vi "box catch.vi"(8 "Error In":errorcluster, 9 "Position in":T4, 11 "main.ctl":T1) -> (0 "Error Out":errorcluster, 1 "Position out":T4, 3 "main.ctl 2":T1={"vision board"={"common room"=[["red", "black", "blue", "", "green"], ["", "", "", "", ""], ["", "", "", "", ""]], "recycle"="NONE"}, "block box"={"block box"=[["", "Black", "", ""], ["", "Red", "", ""], ["Black", "", "", "Blue"]]}, "on robot "=[], "base position"=[], "On robot target"=[]})   [LabVIEW 2019]
uses:
  main data.ctl
  vision/vision_board_ctl.ctl
  block box.ctl
  subVI/move/position cluster.ctl
  box state.ctl
  subVI/move control/move and align/move_cluster.ctl
  servo state.ctl
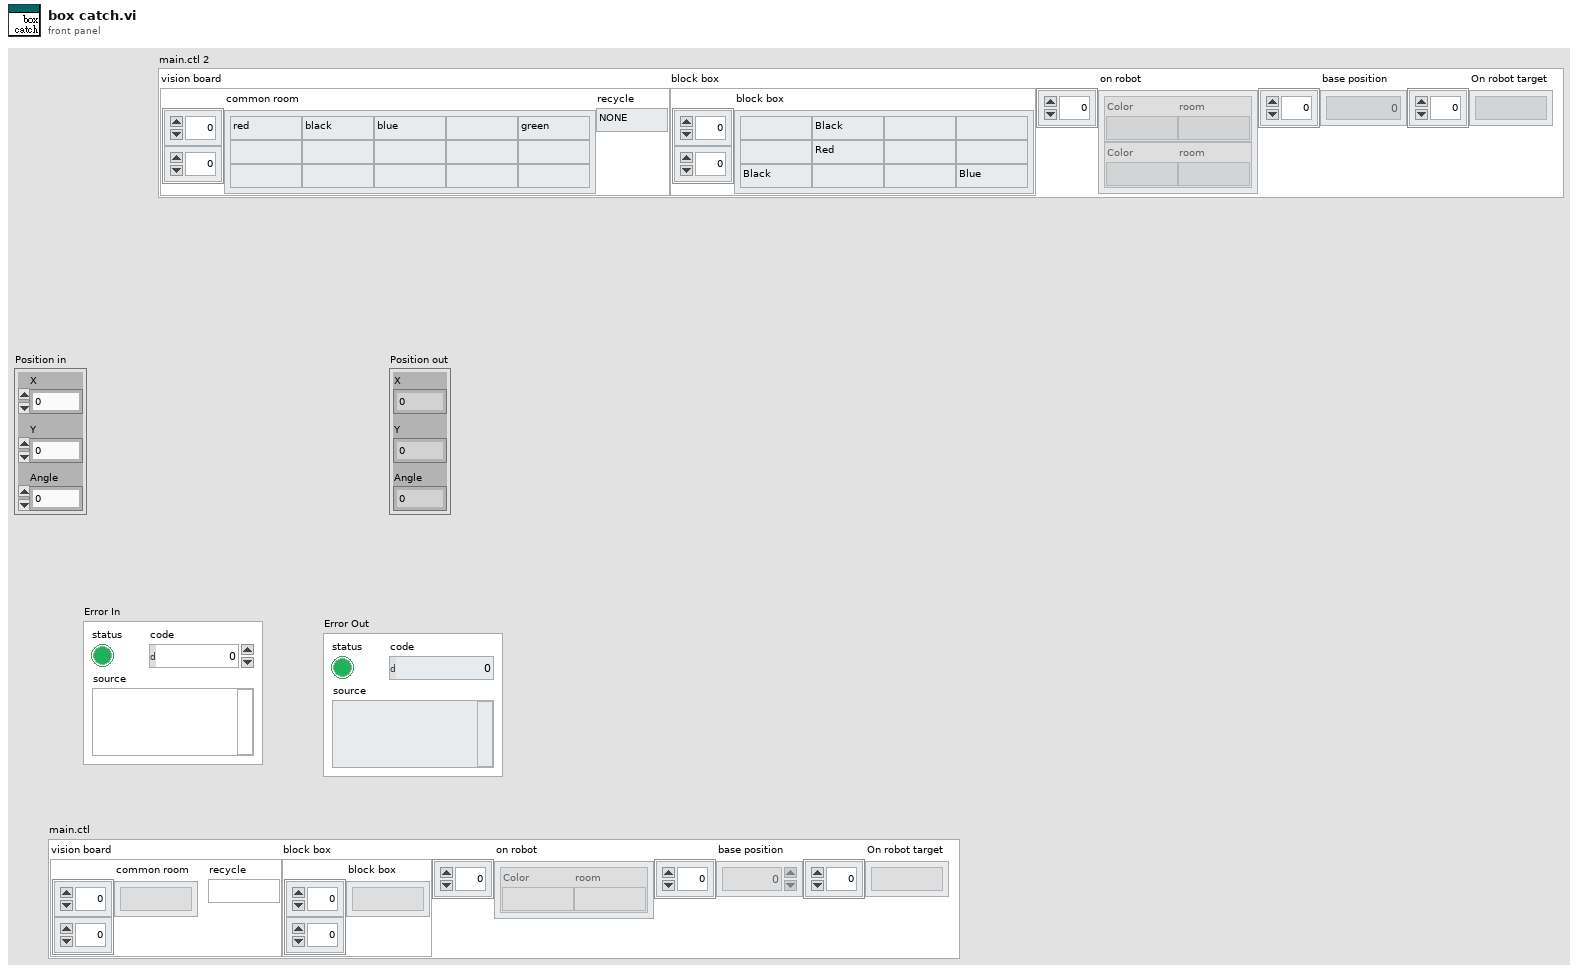
[diagram p1: front panel]
types:
  T1 = typedef "main data.ctl" = cluster{"vision board":T2, "block box":T3, "on robot ":cluster{"Color":string, "room":string}[], "base position":dbl[], "On robot target":string[]}
  T2 = typedef "vision_board_ctl.ctl" = cluster{"common room":string[][], "recycle":string}
  T3 = typedef "block box.ctl" = cluster{"block box":string[][]}
  T4 = typedef "position cluster.ctl" = cluster{"X":dbl, "Y":dbl, "Angle":dbl}
  T5 = typedef "servo state.ctl" = enum16{"catch", "cam-1", "put", "side", "center", "side-2", "put-2"}
  T6 = typedef "move_cluster.ctl" = cluster{"X":dbl, "Y":dbl, "degree":dbl, "speed":dbl}
  T7 = typedef "box state.ctl" = enum16{"init", "vision", "catch"}
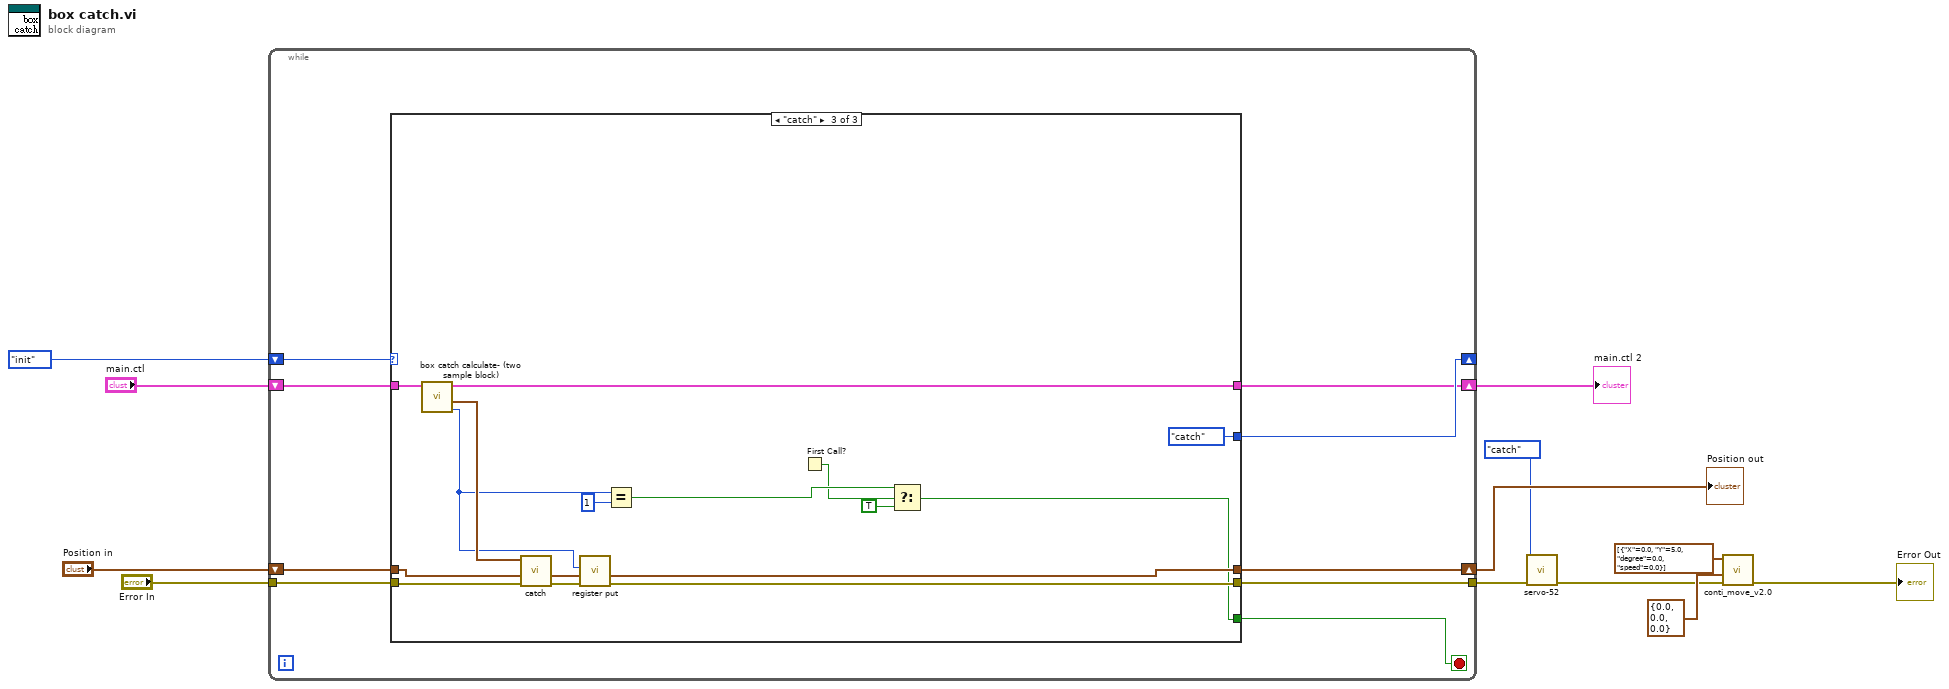
[diagram p0: block diagram]
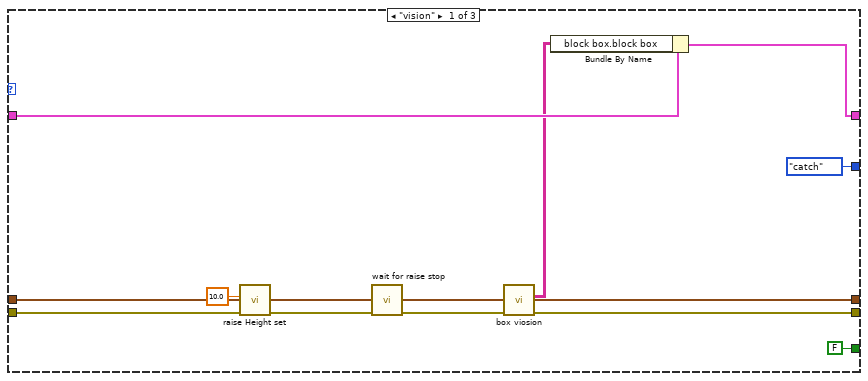
[diagram p2: hidden frame]
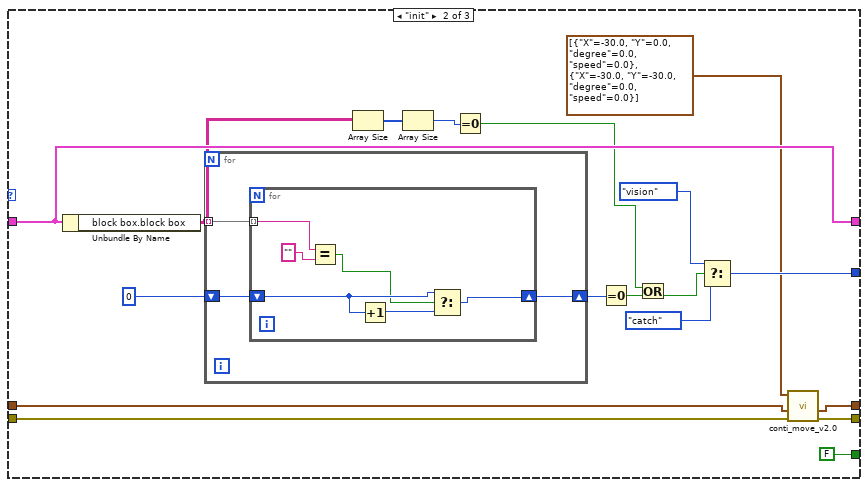
[diagram p3: hidden frame]
diagram:
  n1 = while {
    shift-right: [w19] -> _
    shift-left: box_state."init" -> [w20]
    tunnel: "Error In" -> [w17]
    tunnel: [w16] -> w5
    shift-right: [w13] -> w7
    shift-left: "main.ctl" -> [w21]
    shift-right: [w14] -> w8
    shift-left: "Position in" -> [w15]
    stop <- w18 stop-if-true
    n2 = case shown="\"catch\"" w20 {
      tunnel: w21 -> [w29 w43 w74]
      tunnel: [box_state."catch" ("Enum") w45 box_state."catch" ("Enum")] -> w19
      tunnel: [FALSE FALSE w63] -> w18
      tunnel: w17 -> [w22 w34 w72]
      tunnel: [w30 w36 w68] -> w16
      tunnel: w15 -> [w23 w33 w71]
      tunnel: [w23 w35 w70] -> w14
      tunnel: [w27 w43 w73] -> w13
      frame "vision" {
        n3 = call "raise Height set.vi"("error in (no error)"=w22, "Height_cm"=10.0) -> ("error out"=w25:errorcluster)  [unwired: 9 in]
        n4 = call "wait for raise stop.vi"("Error In"=w25) -> ("Error Out"=w24:errorcluster)  [unwired: 10 in]
        n5 = call "box viosion.vi"("Error In"=w24) -> ("error out"=w30:errorcluster, "Array out"=w28:string[][])  [unwired: 9 in]
        n6 = Bundle By Name(cluster=w29, "block box.block box"=w28) -> (w27:T1)
      }
      frame "init" {
        n7 = Unbundle By Name(w43) -> ("block box.block box"=w41:string[][])
        n8 = for {
          tunnel: w41 -> [w53] mode=indexing
          shift-right: [w51] -> w50
          shift-left: 0 -> [w52]
          n9 = for {
            tunnel: w53 -> [w59] mode=indexing
            shift-right: [w57] -> w51
            shift-left: w52 -> [w55]
            n10 = Equal?(x=w59, y="") -> (x = y?=w54:bool)
            n11 = Increment(x=w55) -> (x+1=w56:i32)
            n12 = Select(t=w55, s=w54, f=w56) -> (s? t:f=w57:i32)
          }
        }
        n13 = Array Size(array=w41) -> (size(s)=w40:i32[])
        n14 = Array Size(array=w40) -> (size(s)=w39:i32)
        n15 = Equal To 0?(x=w39) -> (x = 0?=w38:bool)
        n16 = Equal To 0?(x=w50) -> (x = 0?=w48:bool)
        n17 = Or(x=w38, y=w48) -> (x .or. y?=w42:bool)
        n18 = Select(t=box_state."vision" ("Enum"), s=w42, f=box_state."catch" ("Enum")) -> (s? t:f=w45:T7)
        n19 = call "conti_move_v2.0.vi"("error in (no error)"=w34, "Position"=w33, "route"=T6[] [{"X"=-30.0, "Y"=0.0, "degree"=0.0, "speed"=0.0}, {"X"=-30.0, "Y"=-30.0, "degree"=0.0, "speed"=0.0}]) -> ("error out"=w36:errorcluster, "Position out"=w35:T4)  [unwired: 7 in]
      }
      frame "catch" {
        n20 = call "box catch calculate- (two sample block).vi"("main.ctl"=w74) -> ("register address"=w65:i32, "box position"=w69:cluster{i32, i32}, "output cluster"=w73:T1)  [unwired: 8 in]
        n21 = call "catch.vi"("error in (no error)"=w72, "Position in"=w71, "catch position"=w69) -> ("error out"=w66:errorcluster, "Position out"=w70:T4)  [unwired: 7 in]
        n22 = call "register put.vi"("error in (no error)"=w66, "register address"=w65) -> ("error out"=w68:errorcluster)  [unwired: 9 in]
        n23 = Equal?(x=w65, y=1) -> (x = y?=w62:bool)
        n24 = First Call?() -> (First Call?: T/F=w61:bool)
        n25 = Select(t=w62, s=w61, f=TRUE) -> (s? t:f=w63:bool)
      }
    }
  }
  "Position out" <- w8
  "main.ctl 2" <- w7
  n26 = call "servo-52.vi"("error in (no error)"=w5, "Enum"=servo_state."catch") -> ("error out"=w2:errorcluster)  [unwired: 9 in]
  n27 = call "conti_move_v2.0.vi"("error in (no error)"=w2, "Position"=T4 {"X"=0.0, "Y"=0.0, "Angle"=0.0}, "route"=T6[] [{"X"=0.0, "Y"=5.0, "degree"=0.0, "speed"=0.0}]) -> ("error out"=→"Error Out":errorcluster)  [unwired: 7 in, 1 out]
